vi "Measurement Logic.vi"() -> ()   [LabVIEW 2021, in "Crosstalk_Audio ADC.lvlib"]
uses:
  Crosstalk_Audio ADC.lvlib
  Measurement Configuration.ctl
  <vilib>/MeasurementLink/MeasurementLink Measurement Server/Measure Call Context/Measure Call Context.lvclass
  Measurement Results.ctl
  shared/controls/Sync Commands.ctl
  <vilib>/DAQmx/create/channels.llb/DAQmx Create Channel (AO-FuncGen).vi
  <vilib>/PDM Acquisition Toolkit/host/API/Public/Start/Start PCM Input Task.vi
  <vilib>/PDM Acquisition Toolkit/host/API/Public/Read/Read PCM Input Waveform.vi
  <vilib>/PDM Acquisition Toolkit/host/API/Public/Clear/Clear PCM Input Task.vi
  shared/Audio ADC Shared.lvlib
  <vilib>/PDM Acquisition Toolkit/host/API/PDM Acquisition Toolkit.lvlib
  shared/controls/Audio ADC Controls.lvlib
panel:
  out "measurement results":T1
  out "measure call context out":refnum<class "Measure Call Context.lvclass">
  in  "measure call context in":refnum<class "Measure Call Context.lvclass">
  in  "measurement configuration":T2={"Full scale range"=2.825, "Channel name"="", "Analog source resource name"="", "Frequency"=0.0, "Amplitude"=0.0, "Protocol capture resource name"="", "Data line"=0, "Interferer channel"=0, "Victim channel"=0, "Sample rate"=44100.0, "Measurement duration"=0.1, "Frame sync edge for channel 0"=1, "Channel count per frame"=2, "Channel length"=32, "Bit depth"=24, "Channel 0 offset"=1, "Endiannes"=0, "Data justification"=0, "Frame length"=64, "Frame sync pulse width"=32, "Bit clock edge sync"=1}
  out "error out":errorcluster
  in  "error in":errorcluster
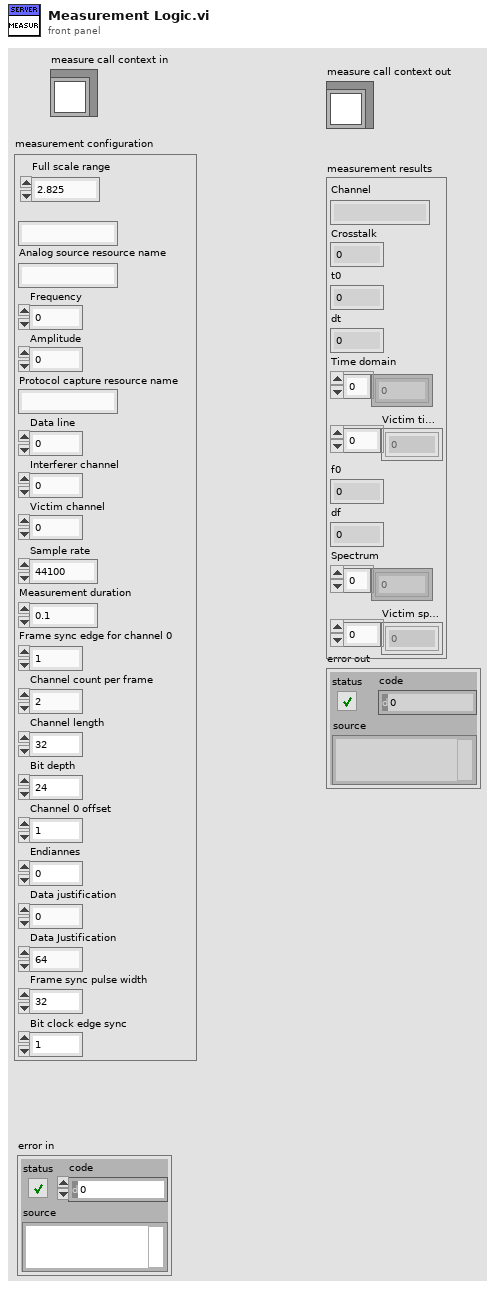
[diagram p1: front panel]
types:
  T1 = typedef "Crosstalk_Audio ADC.lvlib/Measurement Results.ctl" = cluster{"Channel":string, "Crosstalk":dbl, "t0":dbl, "dt":dbl, "Time domain":dbl[], "Victim time domain":dbl[], "f0":dbl, "df":dbl, "Spectrum":dbl[], "Victim spectrum":dbl[]}
  T2 = typedef "Crosstalk_Audio ADC.lvlib/Measurement Configuration.ctl" = cluster{"Full scale range":dbl, "Channel name":string, "Analog source resource name":string, "Frequency":dbl, "Amplitude":dbl, "Protocol capture resource name":string, "Data line":u32, "Interferer channel":u32, "Victim channel":u32, "Sample rate":dbl, "Measurement duration":dbl, "Frame sync edge for channel 0":u32, "Channel count per frame":u32, "Channel length":u32, "Bit depth":u32, "Channel 0 offset":u32, "Endiannes":u32, "Data justification":u32, "Frame length":u32, "Frame sync pulse width":u32, "Bit clock edge sync":u32}
  T3 = typedef "audio adc controls.lvlib/Sync Commands.ctl" = enum16{"NoAction", "GenerationStarted", "AcquisitionCompleted", "GenerationErrored"}
  T4 = typedef "Audio ADC Controls.lvlib/Protocol Settings Dual Channel.ctl" = cluster{"Protocol capture resource name":string, "Data line":u16, "Channel":string, "Clock rate":u32, "Number of words":i32, "Sensitivity":dbl, "Frame sync edge for channel 0":enum32{"Rising", "Falling"}, "Channel count per frame":u8, "Channel length":u16, "Bit depth":u8, "Channel 0 offset":u16, "Endianness":enum32{"MSB First", "LSB First"}, "Data justification":enum32{"Left Justified", "Right Justified"}, "Frame length":u16, "Frame sync pulse width":u16, "Bit clock edge sync":enum32{"Rising", "Falling"}}
  T5 = typedef "PDM Acquisition Class Library.lvlib/PCM Input Task.lvclass/DVR PCM Input Task.ctl" = refnum<data-value>
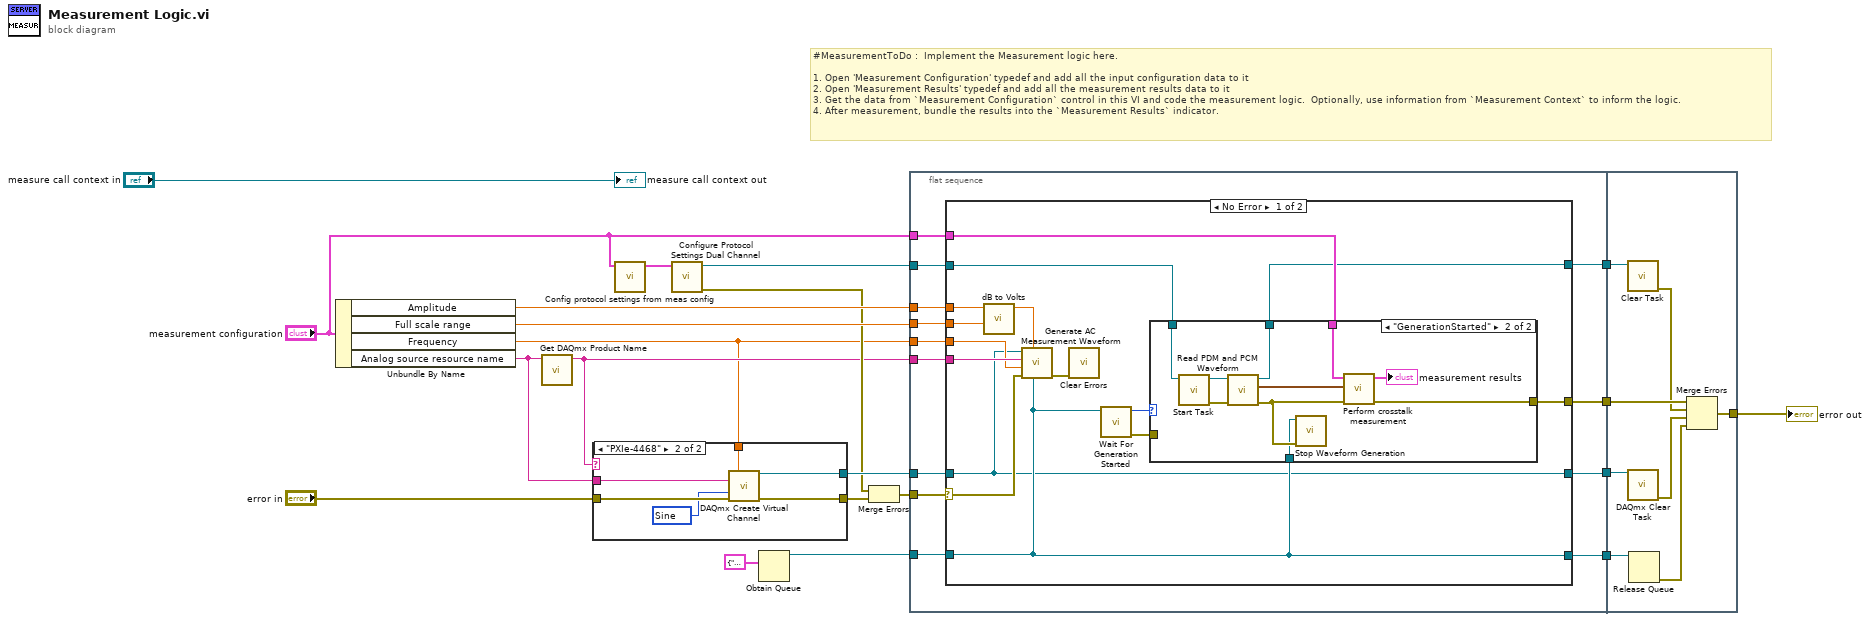
[diagram p0: block diagram]
diagram:
  # "#MeasurementToDo :  Implement the Measurement logic here.\n\n1. Open 'Measurement Configuration' typedef and add all the input configuration data to it\n2. Open 'Measurement Results' typedef and add all the measurement results data to it\n3. Get the data from `Measurement Configuration` control in this VI and code the measurement logic.  Optionally, use information from `Measurement Context` to inform the logic.\n4. After measurement, bundle the results into the `Measurement Results` indicator."
  n1 = Unbundle By Name("measurement configuration") -> ("Amplitude"=w17:dbl, "Full scale range"=w16:dbl, "Frequency"=w2:dbl, "Analog source resource name"=w20:string)
  n2 = call "Get DAQmx Product Name.vi"("DAQmx resource name"=w20) -> ("DAQmx product type"=w3:string)  [unwired: 10 in]
  n3 = case shown="\"PXIe-4468\"" w3 {
    tunnel: w20 -> [_ w27]
    tunnel: "error in" -> [w22 w28]
    tunnel: [w22 w23] -> w13
    tunnel: w2 -> [_ w24]
    tunnel: [_ w25] -> w15
    frame Default {
    }
    frame "PXIe-4468" {
      w26 = 14751 items=["Sine"=14751, "Triangle"=14752, "Square"=14753, "Sawtooth"=14754] ("type")
      n4 = call-poly <vilib>:"DAQmx Create Virtual Channel.vi"("frequency"=w24, "physical channels"=w27, "type"=w26, "error in"=w28) -> ("task out"=w25:refnum<k21>, "error out"=w23:errorcluster)  [unwired: 10 in]
    }
  }
  n5 = call "Config protocol settings from meas config.vi"("measurement configuration"="measurement configuration") -> ("Protocol settings"=w1:T4)  [unwired: 10 in]
  n6 = call "Configure Protocol Settings Dual Channel.vi"("Protocol settings"=w1) -> ("error out"=w12:errorcluster, "PCM input task out"=w14:T5)  [unwired: 9 in]
  n7 = Obtain Queue(element data type=cluster{"Status":T3, "Error":errorcluster} {"Status"=enum."NoAction", "Error"={"status"=FALSE, "code"=0, "source"=""}}) -> (queue out=w4:refnum<queue>)  [unwired: 4 in, 2 out]
  n8 = Merge Errors(w12, w13) -> (w11:errorcluster)
  n9 = flat-sequence {
    tunnel: w17 -> [w41]
    tunnel: w16 -> [w40]
    tunnel: w15 -> [w35]
    tunnel: w4 -> [w31]
    tunnel: w11 -> [w32]
    tunnel: w14 -> [w39]
    tunnel: "measurement configuration" -> [w38]
    tunnel: [w30] -> w9
    tunnel: [w36] -> w8
    tunnel: [w37] -> w7
    tunnel: [w29] -> w6
    tunnel: w3 -> [w34]
    tunnel: w2 -> [w33]
    tunnel: w9 -> [w80]
    tunnel: w8 -> [w79]
    tunnel: w7 -> [w77]
    tunnel: w6 -> [w78]
    tunnel: [w73] -> w5
    frame #0 {
      n10 = case shown="No Error" w32 {
        selector: w32 -> [w44 w71]
        tunnel: w41 -> [w56 _]
        tunnel: w40 -> [w55 _]
        tunnel: w39 -> [w52 w72]
        tunnel: w38 -> [w51 _]
        tunnel: w31 -> [w43 w70]
        tunnel: [w48 w71] -> w37
        tunnel: [w47 w72] -> w36
        tunnel: w35 -> [w42 w69]
        tunnel: w34 -> [w46 _]
        tunnel: w33 -> [w45 _]
        tunnel: [w43 w70] -> w30
        tunnel: [w42 w69] -> w29
        frame No Error {
          n11 = call "dB to Volts.vi"("Full scale range"=w55, "Voltage(dB)"=w56) -> ("Voltage(volts)"=w54:dbl)  [unwired: 9 in]
          n12 = call "Generate AC Measurement Waveform.vi"("hardware commands sync queue"=w43, "Voltage(volts)"=w54, "error in"=w44, "Frequency"=w45, "DAQmx product name"=w46, "DSG task in"=w42) -> ("error out"=w53:errorcluster)  [unwired: 4 in, 1 out]
          n13 = call <vilib>:"Clear Errors.vi"("error in (no error)"=w53) -> ()  [unwired: 5 in, 2 out]
          n14 = call "Wait For Generation Started.vi"("hardware commands sync queue"=w43) -> ("error out"=w49:errorcluster, "Status"=w50:T3)  [unwired: 9 in]
          n15 = case shown="\"GenerationStarted\"" w50 {
            tunnel: w52 -> [w57 w66]
            tunnel: [w58 w62] -> w48
            tunnel: w51 -> [_ w65]
            tunnel: w49 -> [w58 _]
            tunnel: [w57 w60] -> w47
            tunnel: w43 -> [_ w59]
            frame Default {
            }
            frame "GenerationStarted" {
              n16 = call-poly <vilib>:"Start Task.vi"("PCM input task in"=w66) -> ("error out"=w68:errorcluster, "PCM input task out"=w67:T5)  [unwired: 9 in]
              n17 = call-poly <vilib>:"Read PDM and PCM Waveform.vi"("error in"=w68, "PCM input task In"=w67) -> ("error out"=w63:errorcluster, "PCM waveforms"=w64:waveform(dbl)[], "PCM input task out"=w60:T5)  [unwired: 4 in, 3 out]
              n18 = call "Stop Waveform Generation.vi"("error in (no error)"=w63, "Hw sync command Q"=w59) -> ()  [unwired: 10 in]
              n19 = call "Perform crosstalk measurement.vi"("error in (no error)"=w63, "I2S waveforms"=w64, "measurement configuration"=w65) -> ("error out"=w62:errorcluster, "measurement results"=→"measurement results":T1)  [unwired: 7 in]
            }
          }
        }
        frame Error {
        }
      }
    }
    frame #1 {
      n20 = call-poly <vilib>:"Clear Task.vi"("PCM input task in"=w79) -> ("error out"=w76:errorcluster)  [unwired: 10 in]
      n21 = call <vilib>:"DAQmx Clear Task.vi"("task in"=w78) -> ("error out"=w75:errorcluster)  [unwired: 14 in]
      n22 = Release Queue(queue=w80) -> (error out=w74:errorcluster)  [unwired: 2 in, 2 out]
      n23 = Merge Errors(w77, w76, w75, w74) -> (w73:errorcluster)
    }
  }
  "error out" <- w5
  "measure call context out" <- "measure call context in"
